vi "FreshSingleItem.vi"(8 "error in (no error)":errorcluster, 10 "TableItem":refnum<vi>, 11 "MakeTableItem in":refnum<class "ConcreteTableItem.lvclass">) -> (0 "error out":errorcluster, 3 "MakeTableItem out":refnum<class "ConcreteTableItem.lvclass">)   [LabVIEW 2015, in "ActorManagement.lvlib" / "ConcreteTableItem.lvclass"]
uses:
  ConcreteTableItem.lvclass
  ConcreteTableItem.lvclass/ConcreteTableItem.ctl
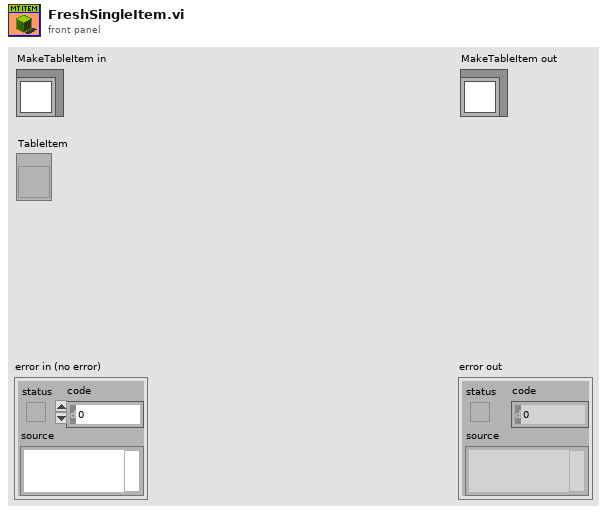
[diagram p1: front panel]
types:
  T1 = cluster{"背景色":u32, "姓名":string, "学号":string, "出勤":bool, "课程表":bool, "请假表":bool}
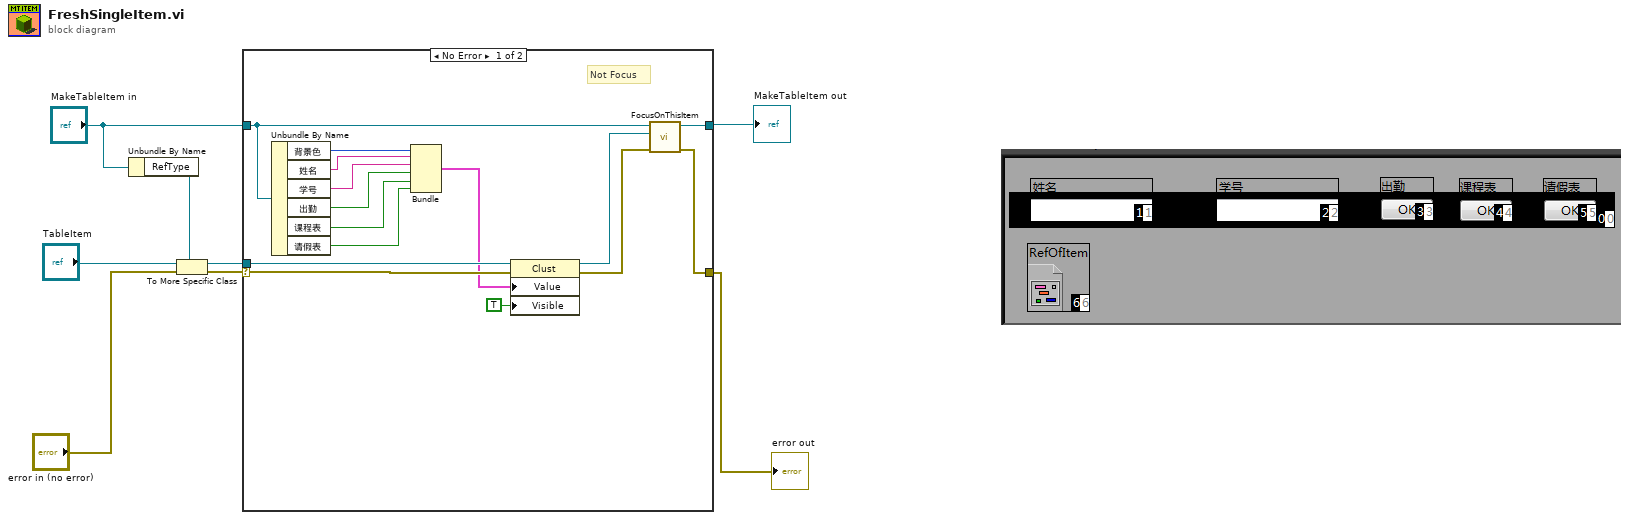
[diagram p0: block diagram]
diagram:
  n1 = Unbundle By Name("MakeTableItem in") -> ("RefType"=w7:refnum<vi>)
  n2 = To More Specific Class(target class=w7, reference="TableItem", error in="error in (no error)") -> (specific class reference=w5:refnum<vi>, error out=w3:errorcluster)
  n3 = case shown="No Error" w3 {
    selector: w3 -> [w22 w24]
    tunnel: "MakeTableItem in" -> [w14 w25]
    tunnel: w5 -> [w23 _]
    tunnel: [w10 w25] -> w2
    tunnel: [w11 w24] -> w1
    frame No Error {
      # "Not Focus"
      n4 = Unbundle By Name(w14) -> ("背景色"=w21:u32, "姓名"=w20:string, "学号"=w19:string, "出勤"=w18:bool, "课程表"=w17:bool, "请假表"=w16:bool)
      n5 = Bundle("背景色"=w21, "姓名"=w20, "学号"=w19, "出勤"=w18, "课程表"=w17, "请假表"=w16) -> (w15:T1)  [unwired: 1 in]
      n6 = property class="Clust"(reference=w23, error in=w22, "Value"=w15, "Visible"=TRUE) -> (reference out=w13:refnum<vi>, error out=w12:errorcluster)
      n7 = call-dynamic "FocusOnThisItem.vi"("error in (no error)"=w12, "ItemCtlRef"=w13, "MakeTableItem in"=w14) -> ("error out"=w11:errorcluster, "MakeTableItem out"=w10:refnum<class "ConcreteTableItem.lvclass">)  [unwired: 7 in]
    }
    frame Error {
    }
  }
  "error out" <- w1
  "MakeTableItem out" <- w2
